vi "Init.vi"(9 "Queue jettl":refnum<class "Queue jettl.lvclass">, 10 "Alias":string) -> (3 "Queue Create Msg Strategy out":refnum<class "Queue Create Msg Strategy.lvclass">)   [LabVIEW 2021, in "jettl.lvlib" / "Queue Create.lvlib" / "Queue Create Msg Strategy.lvclass"]
uses:
  Queue Create Msg Strategy.lvclass
  Queue jettl/Queue jettl.lvclass
  Queue Create Msg Strategy.lvclass/Queue Create Msg Strategy.ctl
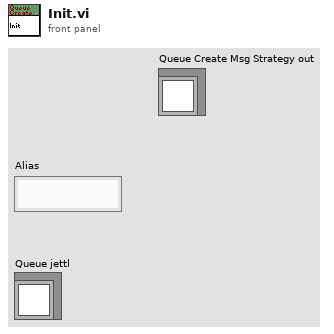
[diagram p1: front panel]
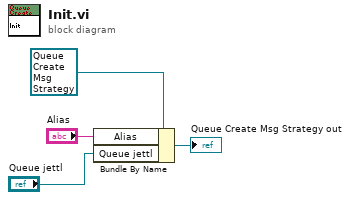
[diagram p0: block diagram]
diagram:
  n1 = Bundle By Name(cluster=refnum<class "Queue Create Msg Strategy.lvclass"> refnum ("Create Msg in"), "Alias"="Alias", "Queue jettl"="Queue jettl") -> (→"Queue Create Msg Strategy out":refnum<class "Queue Create Msg Strategy.lvclass">)
